vi "IAmGLF-NotARefnum.vi"(11 "Test_Button in":refnum<class "Test_Button.lvclass">) -> (2 "Not A Valid Refnum?":bool=TRUE, 3 "Test_Button out":refnum<class "Test_Button.lvclass">)   [LabVIEW 2020, in "Test_Button.lvclass"]
doc: "<B>Summary</B>\nReturns <B>True</B> if the class is invalid."
uses:
  Test_Button.lvclass
  Test_Button.lvclass/Test_Button.ctl
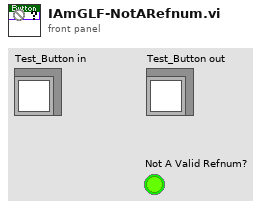
[diagram p1: front panel]
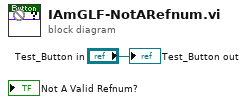
[diagram p0: block diagram]
diagram:
  "Test_Button out" <- "Test_Button in"
